vi "Close Plugin SubPanel.vi"(8 "error in (no error)":errorcluster, 10 "gRPC Port":i32, 11 "CIF_UI in":refnum<class "CIF_UI.lvclass">) -> (0 "error out":errorcluster, 3 "CIF_UI out":refnum<class "CIF_UI.lvclass">)   [LabVIEW 2021, in "CIF_UI.lvclass"]
uses:
  CIF_UI.lvclass
  CIF_UI.lvclass/CIF_UI.ctl
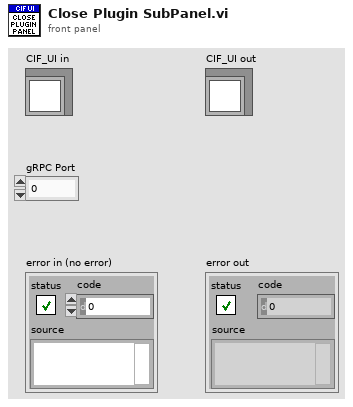
[diagram p1: front panel]
types:
  T1 = typedef "CIF_UI.lvclass/Plugin Subpanel Map.ctl" = map{i32, T2}
  T2 = typedef "CIF_UI.lvclass/Subpanel Data.ctl" = cluster{"VI Reference":refnum<vi>, "Plugin Subpanel Events":T3}
  T3 = typedef "CIF_UI.lvclass/Plugin Subpanel Events.ctl" = cluster{"Plugin Shutdown":refnum<user-event>}
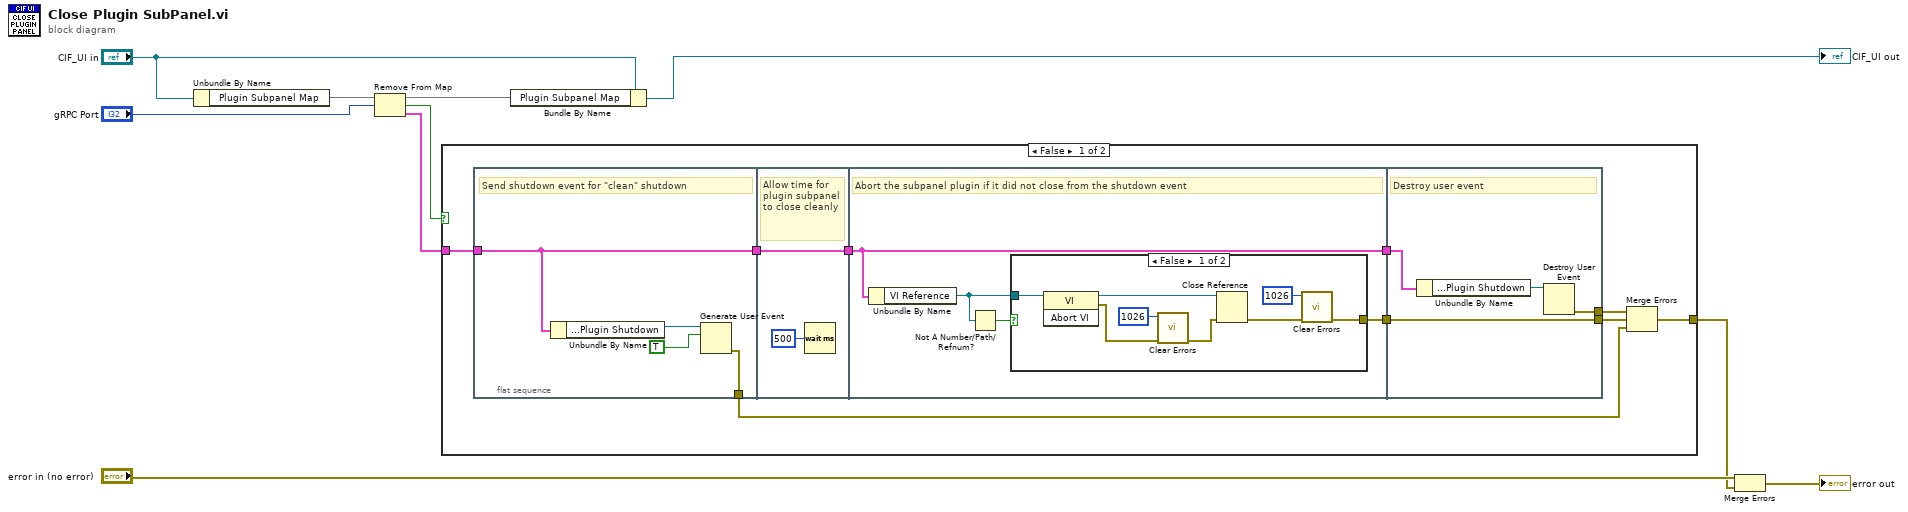
[diagram p0: block diagram]
diagram:
  n1 = Unbundle By Name("CIF_UI in") -> ("Plugin Subpanel Map"=w7:T1)
  n2 = Remove From Map(10:"gRPC Port", 11:w7) -> (1:w5:T2, 2:w4:bool, 3:w2:T1)
  n3 = case shown="False" w4 {
    tunnel: [w11 _] -> w9
    tunnel: w5 -> [w19 _]
    frame False {
      n4 = flat-sequence {
        tunnel: w19 -> [w21]
        tunnel: [w21] -> w17
        tunnel: [w20] -> w12
        tunnel: [w25] -> w18
        tunnel: w17 -> [w25]
        tunnel: w18 -> [w26]
        tunnel: [w29] -> w16
        tunnel: [w26] -> w15
        tunnel: [w41] -> w13
        tunnel: w16 -> [w41]
        tunnel: w15 -> [w40]
        tunnel: [w38] -> w14
        frame #0 {
          # "Send shutdown event for \"clean\" shutdown"
          n5 = Unbundle By Name(w21) -> ("Plugin Subpanel Events.Plugin Shutdown"=w23:refnum<user-event>)
          n6 = Generate User Event(user event=w23, event data cluster=TRUE ("event data")) -> (error out=w20:errorcluster)  [unwired: 2 in, 1 out]
        }
        frame #1 {
          # "Allow time for plugin subpanel to close cleanly"
          n7 = Wait (ms)(milliseconds to wait=u32 500) -> ()  [unwired: 1 out]
        }
        frame #2 {
          # "Abort the subpanel plugin if it did not close from the shutdown event"
          n8 = Unbundle By Name(w26) -> ("VI Reference"=w27:refnum<vi>)
          n9 = Not A Number/Path/Refnum?(number/path/refnum=w27) -> (NaN/Path/Refnum?=w28:bool)
          n10 = case shown="False" w28 {
            tunnel: w27 -> [w37 _]
            tunnel: [w30 _] -> w29
            frame False {
              n11 = invoke class="VI" method="Abort VI"(reference=w37) -> (reference out=w36:refnum<vi>, error out=w34:errorcluster)  [unwired: 2 in, 1 out]
              n12 = call <vilib>:"Clear Errors.vi"("error in (no error)"=w34, "specific error code to clear (0: all)"=1026) -> ("error out"=w33:errorcluster)  [unwired: 4 in, 1 out]
              n13 = Close Reference(reference=w36, error in (no error)=w33) -> (error out=w31:errorcluster)
              n14 = call <vilib>:"Clear Errors.vi"("error in (no error)"=w31, "specific error code to clear (0: all)"=1026) -> ("error out"=w30:errorcluster)  [unwired: 4 in, 1 out]
            }
            frame True {
            }
          }
        }
        frame #3 {
          # "Destroy user event"
          n15 = Unbundle By Name(w40) -> ("Plugin Subpanel Events.Plugin Shutdown"=w39:refnum<user-event>)
          n16 = Destroy User Event(user event=w39) -> (error out=w38:errorcluster)  [unwired: 1 in]
        }
      }
      n17 = Merge Errors(w14, w13, w12) -> (w11:errorcluster)
    }
    frame True {
    }
  }
  n18 = Bundle By Name(cluster="CIF_UI in", "Plugin Subpanel Map"=w2) -> (→"CIF_UI out":refnum<class "CIF_UI.lvclass">)
  n19 = Merge Errors("error in (no error)", w9) -> (→"error out":errorcluster)
